vi "datalogger_byte_array_to_value_converter.vi"(0 "Nmbr_of_datapoints":dbl=128.0, 1 "Array In":u8[](array[numeric]), 2 "CH0 AC couple":bool, 3 "CH1 AC couple":bool, 4 "CH1 multiplier":dbl, 5 "CH0 multiplier":dbl, 6 "CH1 Shift V":dbl, 11 "AC/DC":bool, 12 "CH0 Shift V":dbl) -> (7 "HEXVAL":string, 8 "CH1RMS":dbl, 9 "CH2RMS":dbl, 10 "CH1 Vave":dbl, 13 "CH2 Vave":dbl, 14 "Loop count":dbl, 15 "Voltage":dbl[](graph), 16 "CH1DC":dbl, 17 "Current":dbl[](graph), 18 "mV":dbl, 19 "CH2DC":dbl)   [LabVIEW 2012]
uses:
  <vilib>/measure/madcrms.llb/Basic Averaged DC-RMS for 1 Chan.vi
  <vilib>/measure/NI_MAPro.lvlib
panel:
  out "number of samples":dbl
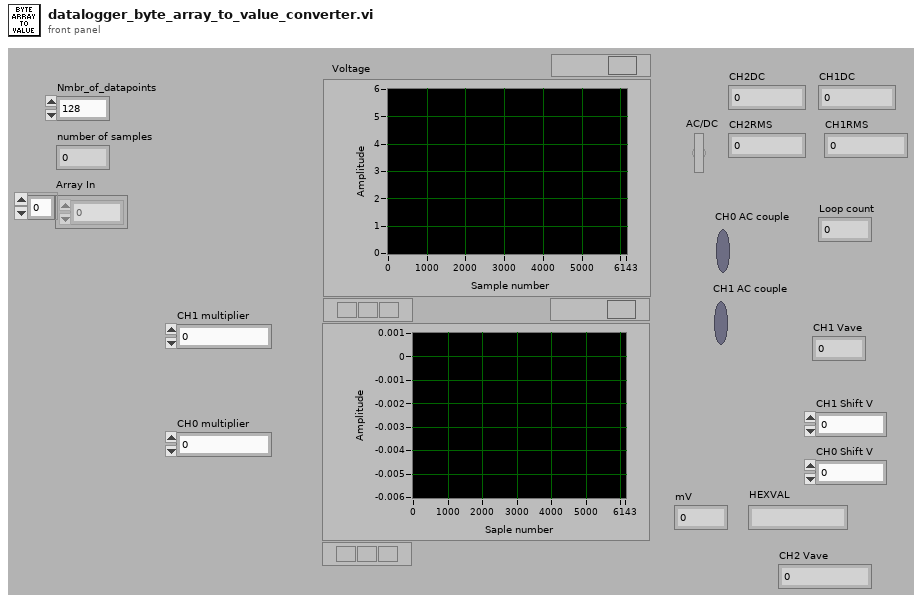
[diagram p1: front panel]
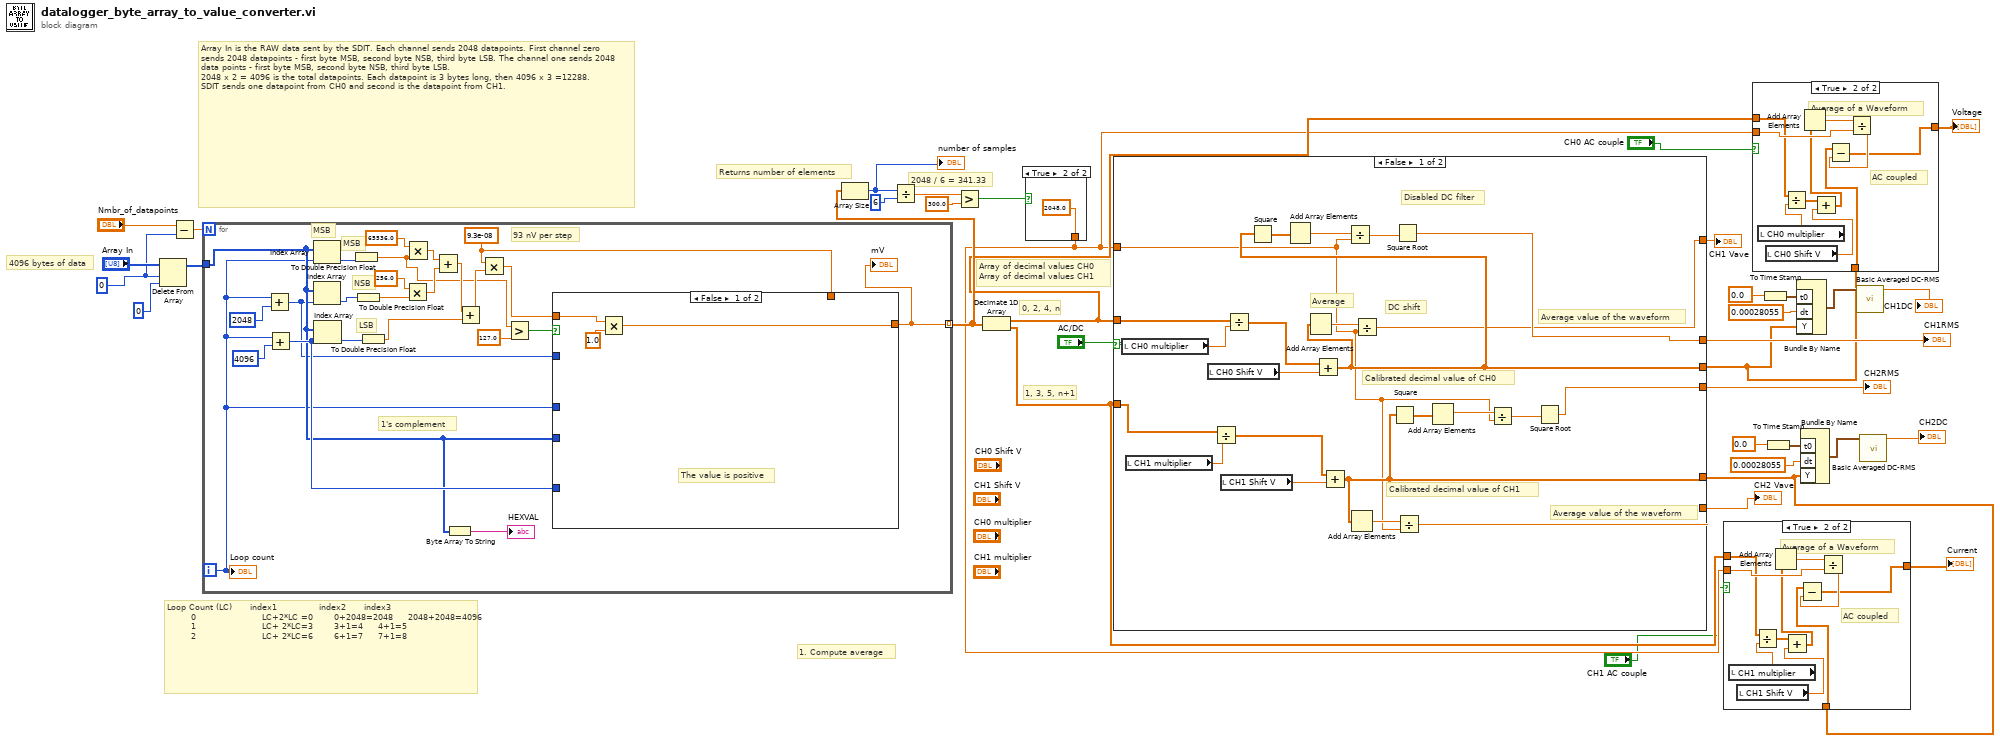
[diagram p0: block diagram]
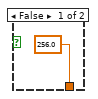
[diagram p4: hidden frame]
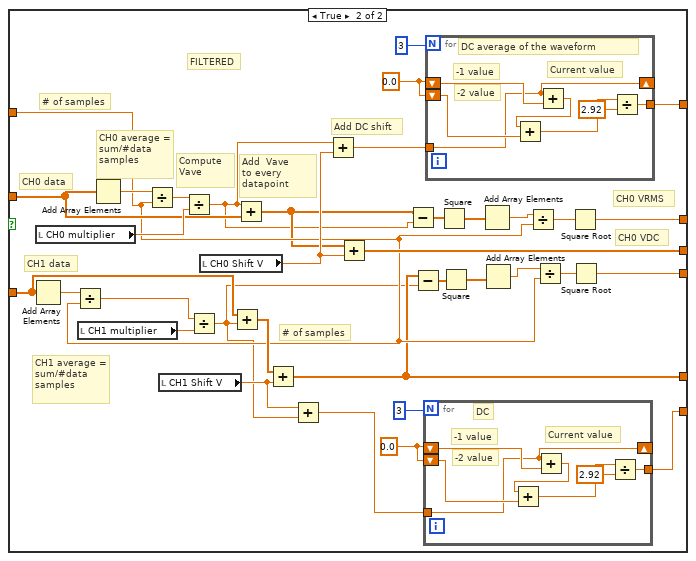
[diagram p5: hidden frame]
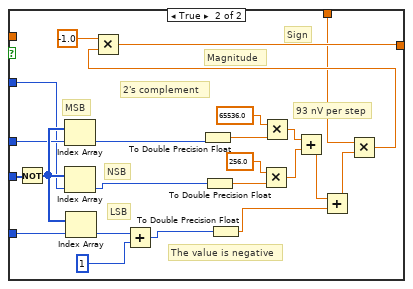
[diagram p6: hidden frame]
diagram:
  w32 = 0
  # "4096 bytes of data"
  # "Array In is the RAW data sent by the SDIT. Each channel sends 2048 datapoints. First channel zero sends 2048 datapoints - first byte MSB, second byte NSB, third byte LSB. The channel one sends 2048 data points - first byte MSB, second byte NSB, third byte LSB.\n2048 x 2 = 4096 is the total datapoints. Each datapoint is 3 bytes long, then 4096 x 3 =12288.\nSDIT sends one datapoint from CH0 and second is the datapoint from CH1."
  # "Returns number of elements"
  # "2048 / 6 = 341.33"
  # "1. Compute average"
  # "1, 3, 5, n+1"
  # "0, 2, 4, n"
  # "Array of decimal values CH0\nArray of decimal values CH1"
  # "Loop Count (LC)      index1              index2      index3      \n        0                      LC+2*LC =0       0+2048=2048     2048+2048=4096\n        1                      LC+ 2*LC=3       3+1=4     4+1=5\n        2                      LC+ 2*LC=6       6+1=7     7+1=8"
  n1 = Delete From Array(array="Array In", length=w32, index=0) -> (array with subset deleted=w31:u8[])  [unwired: 1 out]
  n2 = Subtract(x="Nmbr_of_datapoints", y=w32) -> (x-y=w34:dbl)
  n3 = for {
    N: w34 -> [_]
    tunnel: w31 -> [w42]
    tunnel: [w41] -> w23 mode=indexing
    i -> [w38]
    w45 = 9.3e-08
    # "93 nV per step"
    # "LSB"
    # "MSB"
    # "NSB"
    # "1's complement"
    # "MSB"
    n4 = Add(x=w38, y=2048) -> (x+y=w37:i32)
    n5 = Add(x=w38, y=4096) -> (x+y=w44:i32)
    n6 = Index Array(array=w42, index=w38) -> (element=w48:u8)
    n7 = Index Array(array=w42, index=w37) -> (element=w47:u8)
    n8 = Index Array(array=w42, index=w44) -> (element=w46:u8)
    n9 = To Double Precision Float(number=w48) -> (double precision float=w49:dbl)
    n10 = To Double Precision Float(number=w47) -> (double precision float=w58:dbl)
    n11 = To Double Precision Float(number=w46) -> (double precision float=w54:dbl)
    n12 = Multiply(x=256.0, y=w58) -> (x*y=w56:dbl)
    n13 = Multiply(x=65536.0, y=w49) -> (x*y=w60:dbl)
    n14 = Add(x=w60, y=w56) -> (x+y=w55:dbl)
    n15 = Byte Array To String(unsigned byte array=w42) -> (string=→"HEXVAL":string)
    n16 = Add(x=w55, y=w54) -> (x+y=w53:dbl)
    n17 = Multiply(x=w45, y=w53) -> (x*y=w52:dbl)
    n18 = Greater?(x=w49, y=127.0) -> (0:w51:bool)
    n19 = case shown="False" w51 {
      tunnel: [w63 w86] -> w41
      tunnel: w52 -> [w62 _]
      tunnel: w42 -> [_ w73]
      tunnel: w44 -> [_ w68]
      tunnel: w45 -> [_ w66]
      tunnel: w38 -> [_ w65]
      tunnel: w37 -> [_ w64]
      frame False {
        # "The value is positive"
        n20 = Multiply(x=w62, y=1.0) -> (x*y=w63:dbl)
      }
      frame True {
        # "LSB"
        # "NSB"
        # "The value is negative"
        # "93 nV per step"
        # "Magnitude"
        # "Sign"
        # "2's complement"
        # "MSB"
        n21 = Not(x=w73) -> (.not. x?=w72:u8[])
        n22 = Index Array(array=w72, index=w65) -> (element=w75:u8)
        n23 = Index Array(array=w72, index=w64) -> (element=w74:u8)
        n24 = Index Array(array=w72, index=w68) -> (element=w71:u8)
        n25 = Add(x=w71, y=1) -> (x+y=w69:i32)
        n26 = To Double Precision Float(number=w75) -> (double precision float=w76:dbl)
        n27 = To Double Precision Float(number=w74) -> (double precision float=w82:dbl)
        n28 = To Double Precision Float(number=w69) -> (double precision float=w78:dbl)
        n29 = Multiply(x=256.0, y=w82) -> (x*y=w80:dbl)
        n30 = Multiply(x=65536.0, y=w76) -> (x*y=w84:dbl)
        n31 = Add(x=w84, y=w80) -> (x+y=w79:dbl)
        n32 = Add(x=w79, y=w78) -> (x+y=w77:dbl)
        n33 = Multiply(x=w66, y=w77) -> (x*y=w67:dbl)
        n34 = Multiply(x=-1.0, y=w67) -> (x*y=w86:dbl)
      }
    }
    "mV" <- w41
    "Loop count" <- w38
  }
  n35 = Array Size(array=w23) -> (size(s)=w27:i32)
  "number of samples" <- w27
  n36 = Divide(x=w27, y=6) -> (x/y=w26:dbl)
  n37 = Greater?(x=w26, y=300.0) -> (0:w24:bool)
  n38 = Decimate 1D Array(w23) -> (w6:dbl[], w5:dbl[])
  n39 = case shown="True" w24 {
    tunnel: [256.0 2048.0] -> w4
    frame False {
    }
    frame True {
    }
  }
  n40 = case shown="False" "AC/DC" {
    tunnel: w6 -> [w103 w130]
    tunnel: w5 -> [w111 w129]
    tunnel: [w94 w118] -> w1
    tunnel: [w95 w126] -> w8
    tunnel: [w90 w133] -> w29
    tunnel: [w91 w138] -> w28
    tunnel: w4 -> [w92 w121]
    tunnel: [w102 w113] -> w11
    tunnel: [w96 w112] -> w10
    frame False {
      # "Average value of the waveform"
      # "Average value of the waveform"
      # "Disabled DC filter"
      # "Calibrated decimal value of CH1"
      # "Calibrated decimal value of CH0"
      # "DC shift"
      # "Average"
      n41 = local read "CH0 multiplier"() -> (w106:dbl)
      n42 = local read "CH1 multiplier"() -> (w110:dbl)
      n43 = local read "CH0 Shift V"() -> (w105:dbl)
      n44 = Divide(x=w111, y=w110) -> (x/y=w97:dbl[])
      n45 = local read "CH1 Shift V"() -> (w109:dbl)
      n46 = Divide(x=w103, y=w106) -> (x/y=w108:dbl[])
      n47 = Add(x=w108, y=w105) -> (x+y=w95:dbl[])
      n48 = Square(x=w95) -> (x^2=w104:dbl[])
      n49 = Add Array Elements(numeric array=w104) -> (sum=w89:dbl)
      n50 = Add Array Elements(numeric array=w95) -> (sum=w107:dbl)
      n51 = Add(x=w97, y=w109) -> (x+y=w94:dbl[])
      n52 = Divide(x=w89, y=w92) -> (x/y=w101:dbl)
      n53 = Add Array Elements(numeric array=w94) -> (sum=w93:dbl)
      n54 = Divide(x=w107, y=w92) -> (x/y=w91:dbl)
      n55 = Square(x=w94) -> (x^2=w100:dbl[])
      n56 = Square Root(x=w101) -> (sqrt(x)=w102:dbl)
      n57 = Divide(x=w93, y=w92) -> (x/y=w90:dbl)
      n58 = Add Array Elements(numeric array=w100) -> (sum=w98:dbl)
      n59 = Divide(x=w98, y=w92) -> (x/y=w99:dbl)
      n60 = Square Root(x=w99) -> (sqrt(x)=w96:dbl)
    }
    frame True {
      w135 = 0.0
      w140 = 0.0
      # "FILTERED"
      # "CH1 average = sum/#data samples"
      # "CH0 VRMS"
      # "CH0 VDC"
      # "Add DC shift"
      # "Compute Vave"
      # "# of samples"
      # "# of samples"
      # "CH1 data"
      # "CH0 data"
      # "Add  Vave\nto every datapoint"
      # "CH0 average = sum/#data samples"
      n61 = Add Array Elements(numeric array=w129) -> (sum=w145:dbl)
      n62 = local read "CH0 multiplier"() -> (w142:dbl)
      n63 = Divide(x=w145, y=w121) -> (x/y=w144:dbl)
      n64 = local read "CH1 multiplier"() -> (w141:dbl)
      n65 = Add Array Elements(numeric array=w130) -> (sum=w146:dbl)
      n66 = Divide(x=w146, y=w121) -> (x/y=w119:dbl)
      n67 = local read "CH1 Shift V"() -> (w132:dbl)
      n68 = Divide(x=w119, y=w142) -> (x/y=w116:dbl)
      n69 = Divide(x=w144, y=w141) -> (x/y=w117:dbl)
      n70 = local read "CH0 Shift V"() -> (w137:dbl)
      n71 = Add(x=w129, y=w117) -> (x+y=w143:dbl[])
      n72 = Add(x=w116, y=w130) -> (x+y=w120:dbl[])
      n73 = Add(x=w143, y=w132) -> (x+y=w118:dbl[])
      n74 = Add(x=w132, y=w117) -> (x+y=w131:dbl)
      n75 = Add(x=w116, y=w137) -> (x+y=w136:dbl)
      n76 = Add(x=w120, y=w137) -> (x+y=w126:dbl[])
      n77 = Subtract(x=w120, y=w116) -> (x-y=w114:dbl[])
      n78 = Subtract(x=w118, y=w117) -> (x-y=w115:dbl[])
      n79 = for {
        N: 3 -> [_]
        shift-right: [w147] -> _
        shift-left: w135 -> [w153]
        shift-left: w135 -> [w150]
        tunnel: [w148] -> w133
        tunnel: w131 -> [w147]
        # "DC"
        # "-2 value"
        # "-1 value"
        # "Current value"
        n80 = Add(x=w147, y=w153) -> (x+y=w151:dbl)
        n81 = Add(x=w151, y=w150) -> (x+y=w149:dbl)
        n82 = Divide(x=w149, y=2.92) -> (x/y=w148:dbl)
      }
      n83 = for {
        N: 3 -> [_]
        shift-right: [w154] -> _
        shift-left: w140 -> [w160]
        shift-left: w140 -> [w157]
        tunnel: [w155] -> w138
        tunnel: w136 -> [w154]
        # "DC average of the waveform"
        # "-2 value"
        # "-1 value"
        # "Current value"
        n84 = Add(x=w154, y=w160) -> (x+y=w158:dbl)
        n85 = Add(x=w158, y=w157) -> (x+y=w156:dbl)
        n86 = Divide(x=w156, y=2.92) -> (x/y=w155:dbl)
      }
      n87 = Square(x=w114) -> (x^2=w125:dbl[])
      n88 = Square(x=w115) -> (x^2=w122:dbl[])
      n89 = Add Array Elements(numeric array=w125) -> (sum=w127:dbl)
      n90 = Add Array Elements(numeric array=w122) -> (sum=w123:dbl)
      n91 = Divide(x=w127, y=w121) -> (x/y=w128:dbl)
      n92 = Divide(x=w123, y=w121) -> (x/y=w124:dbl)
      n93 = Square Root(x=w128) -> (sqrt(x)=w113:dbl)
      n94 = Square Root(x=w124) -> (sqrt(x)=w112:dbl)
    }
  }
  "CH2 Vave" <- w29
  "CH1 Vave" <- w28
  "CH1RMS" <- w11
  "CH2RMS" <- w10
  n95 = case shown="True" "CH1 AC couple" {
    tunnel: w1 -> [w161 w171]
    tunnel: w4 -> [_ w170]
    tunnel: [w161 w167] -> w2
    tunnel: w5 -> [_ w165]
    frame False {
      # "DC coupled"
    }
    frame True {
      # "AC coupled"
      # "Average of a Waveform"
      n96 = local read "CH1 multiplier"() -> (w164:dbl)
      n97 = local read "CH1 Shift V"() -> (w163:dbl)
      n98 = Divide(x=w165, y=w164) -> (x/y=w166:dbl[])
      n99 = Add(x=w166, y=w163) -> (x+y=w162:dbl[])
      n100 = Add Array Elements(numeric array=w162) -> (sum=w169:dbl)
      n101 = Divide(x=w169, y=w170) -> (x/y=w168:dbl)
      n102 = Subtract(x=w171, y=w168) -> (x-y=w167:dbl[])
    }
  }
  "Current" <- w2
  n103 = case shown="True" "CH0 AC couple" {
    tunnel: w8 -> [w172 w182]
    tunnel: w4 -> [_ w181]
    tunnel: [w172 w178] -> w7
    tunnel: w6 -> [_ w176]
    frame False {
      # "DC coupled"
    }
    frame True {
      # "AC coupled"
      # "Average of a Waveform"
      n104 = local read "CH0 multiplier"() -> (w175:dbl)
      n105 = local read "CH0 Shift V"() -> (w174:dbl)
      n106 = Divide(x=w176, y=w175) -> (x/y=w177:dbl[])
      n107 = Add(x=w177, y=w174) -> (x+y=w173:dbl[])
      n108 = Add Array Elements(numeric array=w173) -> (sum=w180:dbl)
      n109 = Divide(x=w180, y=w181) -> (x/y=w179:dbl)
      n110 = Subtract(x=w182, y=w179) -> (x-y=w178:dbl[])
    }
  }
  "Voltage" <- w7
  n111 = To Time Stamp(1:0.0 ("t0")) -> (0:w20:timestamp)
  n112 = To Time Stamp(1:0.0 ("t0")) -> (0:w16:timestamp)
  n113 = Bundle By Name("t0"=w20, "dt"=0.00028055, "Y"=w8) -> (w21:waveform(dbl))  [unwired: 1 in]
  n114 = Bundle By Name("t0"=w16, "dt"=0.00028055, "Y"=w1) -> (w17:waveform(dbl))  [unwired: 1 in]
  n115 = call-poly <vilib>:"Basic Averaged DC-RMS.vi"("signal in"=w21) -> ("DC value"=→"CH1DC":dbl)  [unwired: 7 in, 3 out]
  n116 = call-poly <vilib>:"Basic Averaged DC-RMS.vi"("signal in"=w17) -> ("DC value"=→"CH2DC":dbl)  [unwired: 7 in, 3 out]
